vi "words_to_mp3.vi"() -> ()   [LabVIEW 2015]
panel:
  in  "name":string
  in  "words":string
  out "output_words":string
  out "error out 2":errorcluster
  out "Standard Error":string
  out "Return Code":i32
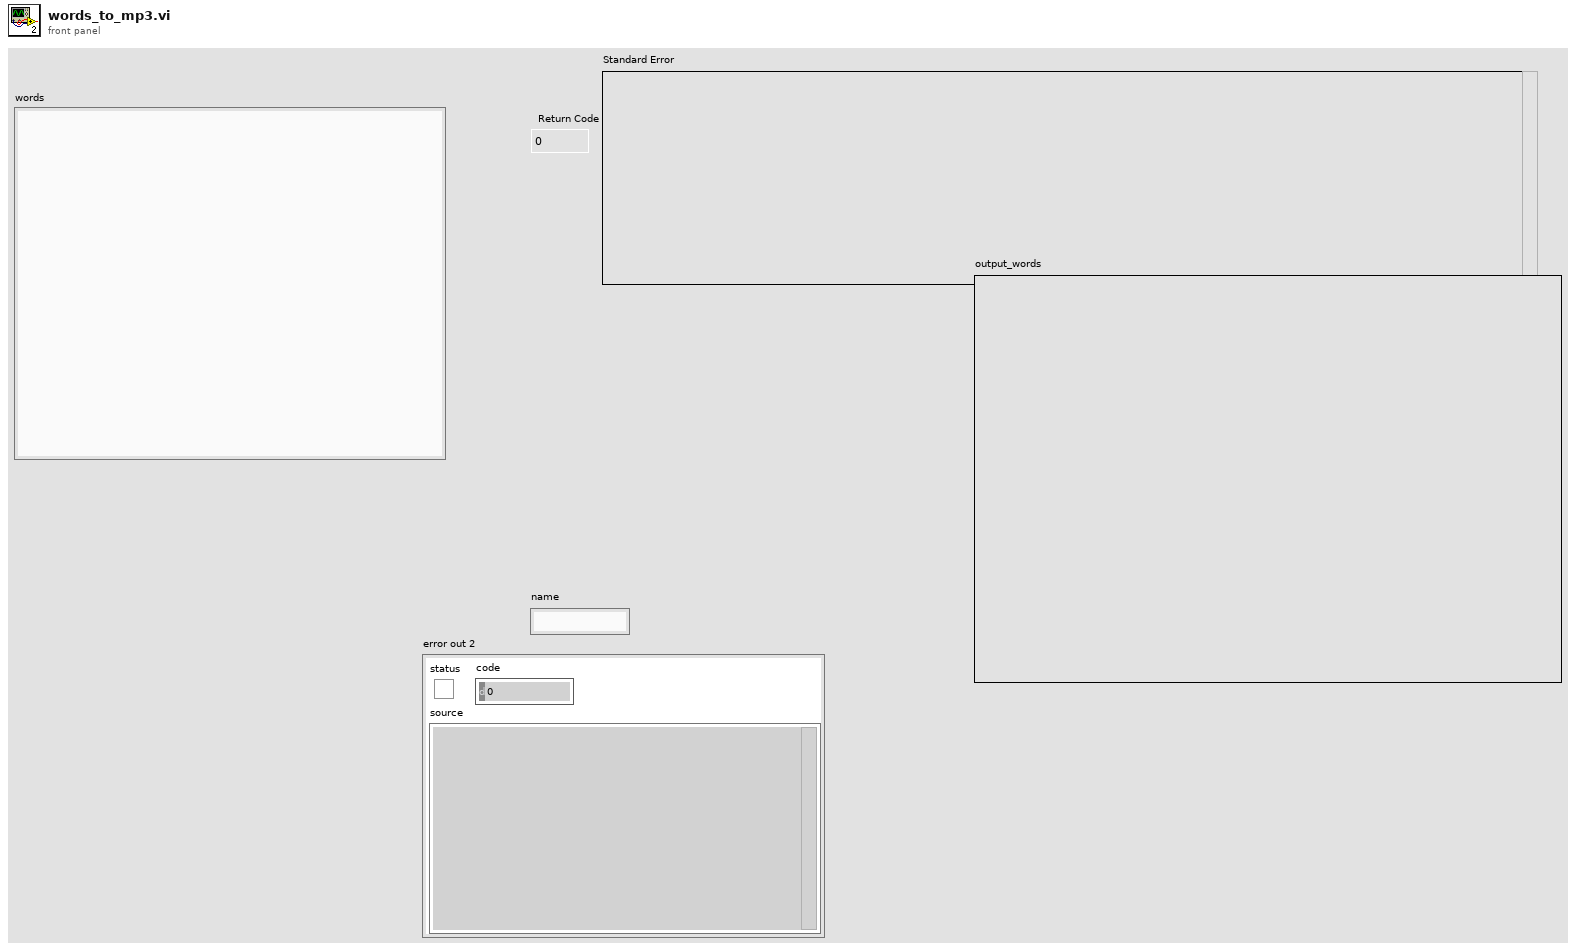
[diagram p1: front panel]
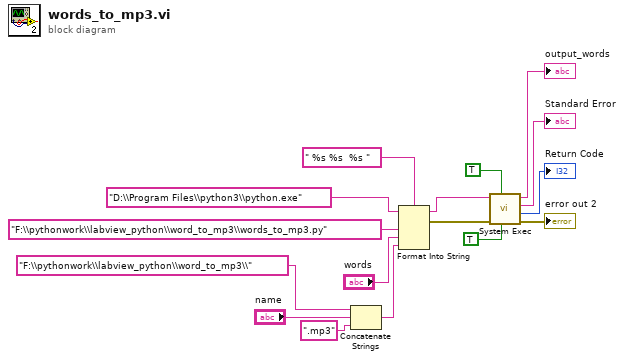
[diagram p0: block diagram]
diagram:
  n1 = Concatenate Strings("F:\\pythonwork\\labview_python\\word_to_mp3\\", "name", ".mp3") -> (w2:string)
  n2 = Format Into String(format string=" %s %s  %s ", initial string="D:\\Program Files\\python3\\python.exe" ("Path to Function"), "F:\\pythonwork\\labview_python\\word_to_mp3\\words_to_mp3.py" ("Path to Function"), "words", w2) -> (resulting string=w13:string, error out=w11:errorcluster)  [unwired: 1 in]
  n3 = call <vilib>:"System Exec.vi"("run minimized? (F)"=TRUE, "wait until completion? (T)"=TRUE, "error in (no error)"=w11, "command line"=w13) -> ("error out"=→"error out 2":errorcluster, "return code"=→"Return Code":i32, "standard error"=→"Standard Error":string, "standard output"=→"output_words":string)  [unwired: 4 in]
